vi "BasicHostExample.vi"() -> ()   [LabVIEW 2015]
uses:
  <vilib>/FPGAPlugInAG/sbRIO-9607/niLvFpga_Open_sbRIO-9607.vi
  <vilib>/rvi/interface/common/dynamic/niFpgaDynamicAddResources.vi
  <vilib>/Utility/error.llb/Error Cluster From Error Code.vi
  <vilib>/rvi/errors/niLvFpgaAdjustHostInterfaceError.vi
  <vilib>/FPGAPlugInAG/Dynamic/niLvFpga_Close_Dynamic.vi
  <vilib>/rvi/interface/nirviOpenFPGA/nirviOpenFPGA.xnode
  Bitfiles/QuadEncdev_FPGATarget_QuadEncTestHarne_guV8O2qA8IY.lvbitx
  QuadEncTestHarness.vi
  <vilib>/rvi/interface/nirviReadWriteControl/nirviReadWriteControl.xnode
  <vilib>/rvi/interface/nirviCloseFPGA/nirviCloseFPGA.xnode
  <vilib>/rvi/interface/Simulation/niFpgaSimulationCallBeginRW.vi
  QuadEncInterface/QuadEncInterface.lvlib
  NiFpgaLv.dll
panel:
  out "CW_direction":bool
  out "RevPosition":i32
  out "AbsPosition":i32
  in  "stop":bool
  out "Output":T1
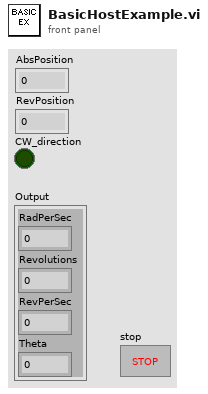
[diagram p1: front panel]
types:
  T1 = cluster{"RadPerSec":sgl, "Revolutions":sgl, "RevPerSec":sgl, "Theta":sgl}
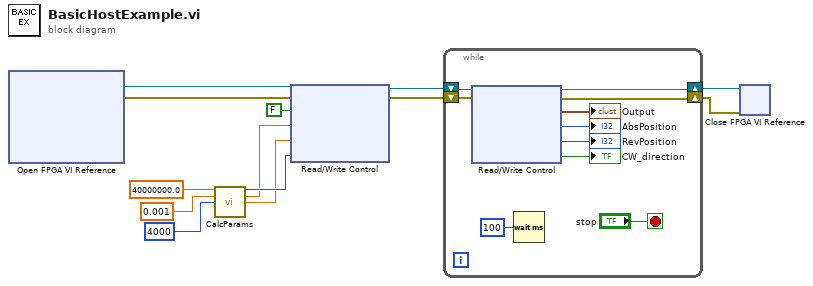
[diagram p0: block diagram]
diagram:
  n1 = xnode "Open FPGA VI Reference"() -> ("FPGA VI Reference Out"=w13:refnum<k20>, "error out"=w12:errorcluster)  [unwired: 2 in]
  n2 = call "CalcParams.vi"("ClkRate"=40000000.0, "dT"=0.001, "TicksPerRev"=u32 4000) -> ("dT"=w7:u32, "dTPerSec"=w6:dbl, "RevPerPulse"=w5:dbl)  [unwired: 10 in]
  n3 = xnode "Read/Write Control"("FPGA VI Reference In"=w13, "error in"=w12, "ReversePolarity"=FALSE, "dTPerSec"=w6, "RevPerPulse"=w5, "dT"=w7) -> ("FPGA VI Reference Out"=w4:refnum<k20>, "error out"=w3:errorcluster)
  n4 = while {
    shift-right: [w19] -> w2
    shift-left: w4 -> [w22]
    shift-right: [w18] -> w1
    shift-left: w3 -> [w23]
    stop <- "stop" stop-if-true
    n5 = xnode "Read/Write Control"("FPGA VI Reference In"=w22, "error in"=w23) -> ("FPGA VI Reference Out"=w19:refnum<k20>, "error out"=w18:errorcluster, "Output"=→"Output":T1, "AbsPosition"=→"AbsPosition":i32, "RevPosition"=→"RevPosition":i32, "CW_direction"=→"CW_direction":bool)
    n6 = Wait (ms)(milliseconds to wait=u32 100) -> ()  [unwired: 1 out]
  }
  n7 = xnode "Close FPGA VI Reference"("FPGA VI Reference In"=w2, "error in"=w1) -> ()  [unwired: 1 out]
